vi "Get Optimization Grid Constants.vi"(11 "Generic Optimization in":refnum<class "Generic Optimization.lvclass">) -> (1 "Bus by ID":T1[](array[typedef]), 2 "Network Data":T3[](array[typedef]), 3 "Generic Optimization out":refnum<class "Generic Optimization.lvclass">)   [LabVIEW 2018, in "Generic Optimization Actor.lvlib" / "Generic Optimization.lvclass"]
uses:
  Generic Optimization.lvclass
  C:/Users/Administrator/Desktop/2018LabVIEW EMS/EMS Generic Actor/EMS Generic/EMS Generic.lvclass
  Optimization Controls/Electrical Network Optimization Data.ctl
  Optimization Controls/Bus by ID.ctl
  <vilib>/ORNL/CSEISMIC DDS/CSEISMIC DDS Base/Data Types/Controls/DeviceID.ctl
  EMS Generic Actor/EMS Generic/EMS Generic.lvclass
  <vilib>/ORNL/CSEISMIC DDS/CSEISMIC DDS Base/CSEISMIC DDS.lvclass
panel:
  out "error out":errorcluster
  in  "error in":errorcluster
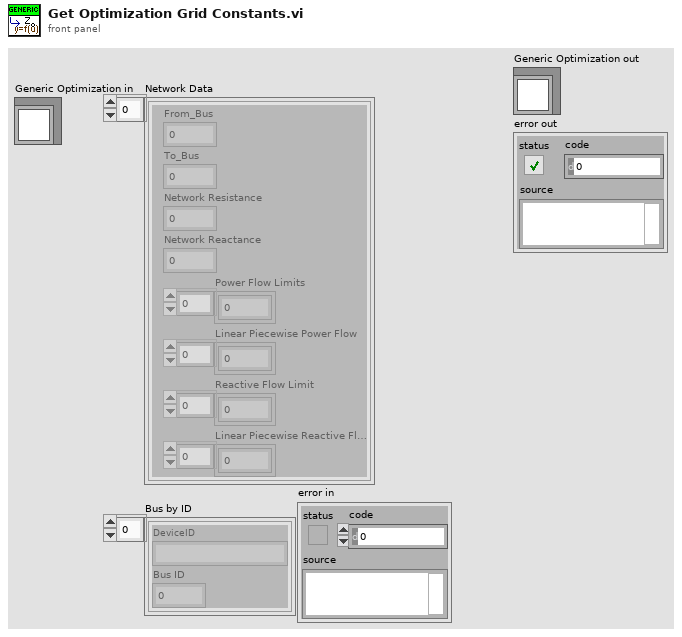
[diagram p1: front panel]
types:
  T1 = typedef "Generic Optimization Actor.lvlib/Generic Optimization.lvclass/Bus by ID.ctl" = cluster{"DeviceID":T2, "Bus ID":dbl}
  T2 = typedef "CSEISMIC DDS.lvlib/CSEISMIC DDS.lvclass/DeviceID.ctl" = string
  T3 = typedef "Generic Optimization Actor.lvlib/Generic Optimization.lvclass/Electrical Network Optimization Data.ctl" = cluster{"From_Bus":dbl, "To_Bus":dbl, "Network Resistance":dbl, "Network Reactance":dbl, "Power Flow Limits":dbl[], "Linear Piecewise Power Flow":dbl[], "Reactive Flow Limit":dbl[], "Linear Piecewise Reactive Flow":dbl[]}
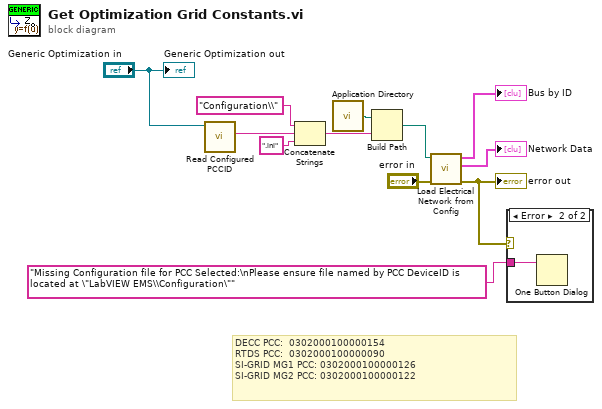
[diagram p0: block diagram]
diagram:
  # "DECC PCC:  0302000100000154\nRTDS PCC:  0302000100000090\nSI-GRID MG1 PCC: 0302000100000126\nSI-GRID MG2 PCC: 0302000100000122"
  n1 = call "Read Configured PCCID.vi"("EMS Generic in"="Generic Optimization in") -> ("PCCID"=w1:T2)  [unwired: 8 in, 2 out]
  n2 = Concatenate Strings("Configuration\\" ("string"), w1, ".ini" ("string")) -> (w9:string)
  n3 = call <vilib>:"Application Directory.vi"() -> ("Application Directory"=w12:path)
  n4 = Build Path(base path=w12, name or relative path=w9) -> (appended path=w8:path)
  n5 = call "Load Electrical Network from Config.vi"("error in"="error in", "configuration file path"=w8) -> ("error out"=w4:errorcluster, "NetworkData"=→"Network Data":T3[], "BusData"=→"Bus by ID":T1[])  [unwired: 7 in]
  "error out" <- w4
  n6 = case shown="Error" w4 {
    tunnel: "Missing Configuration file for PCC Selected:\nPlease ensure file named by PCC DeviceID is located at \"LabVIEW EMS\\Configuration\"" ("message") -> [_ w13]
    frame No Error {
    }
    frame Error {
      n7 = One Button Dialog(message=w13) -> ()  [unwired: 1 in, 1 out]
    }
  }
  "Generic Optimization out" <- "Generic Optimization in"
